vi "LoadCellDAQ.vi"(8 "error in (no error)":errorcluster, 9 "Message Notifiers":T1, 10 "UI Queue":refnum<queue>, 11 "Logging Queue":refnum<queue>) -> (0 "error out":errorcluster)   [LabVIEW 2018]
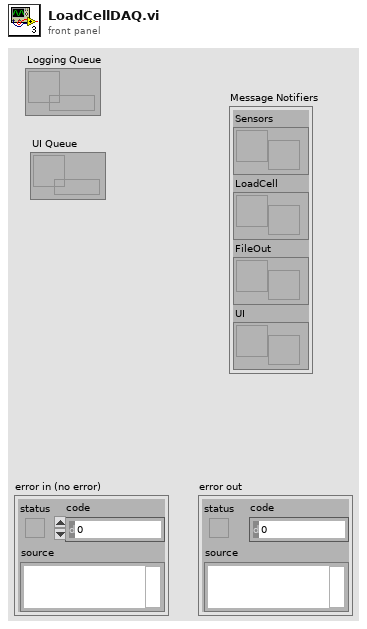
[diagram p1: front panel]
types:
  T1 = cluster{"Sensors":refnum<notifier>, "LoadCell":refnum<notifier>, "FileOut":refnum<notifier>, "UI":refnum<notifier>}
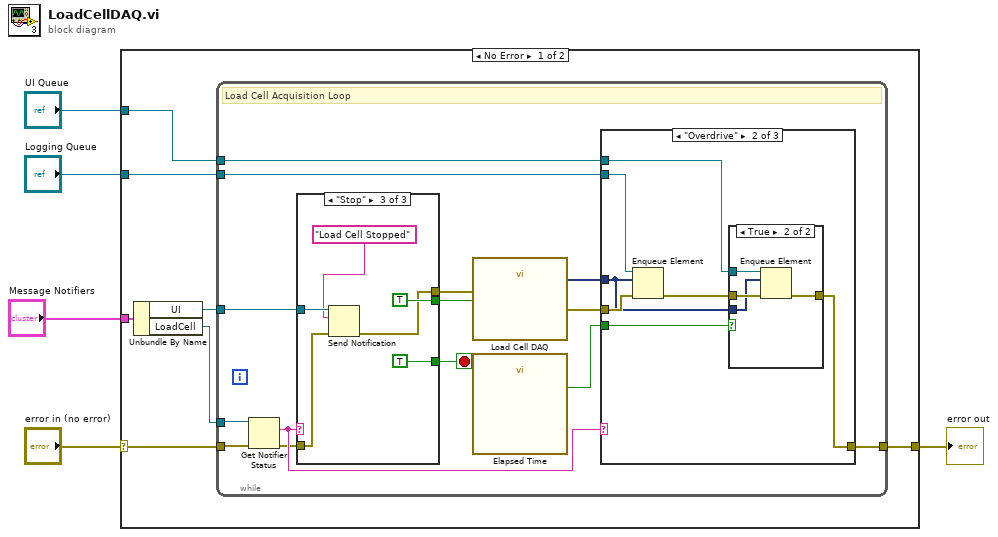
[diagram p0: block diagram]
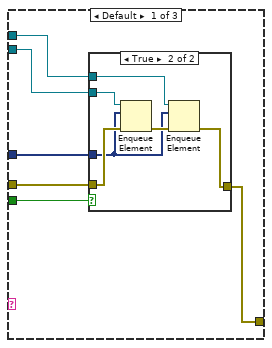
[diagram p2: hidden frame]
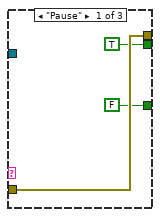
[diagram p6: hidden frame]
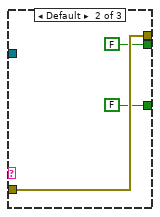
[diagram p7: hidden frame]
diagram:
  n1 = case shown="No Error" "error in (no error)" {
    selector: "error in (no error)" -> [w10 w65]
    tunnel: "Message Notifiers" -> [w12 _]
    tunnel: [w6 w65] -> w4
    tunnel: "Logging Queue" -> [w8 _]
    tunnel: "UI Queue" -> [w7 _]
    frame No Error {
      n2 = Unbundle By Name(w12) -> ("UI"=w11:refnum<notifier>, "LoadCell"=w9:refnum<notifier>)
      n3 = while {
        tunnel: w11 -> [w23]
        tunnel: w10 -> [w13]
        tunnel: w9 -> [w14]
        tunnel: w8 -> [w19]
        tunnel: w7 -> [w18]
        tunnel: [w21] -> w6
        stop <- w24 stop-if-true
        # "Load Cell Acquisition Loop"
        n4 = Get Notifier Status(notifier=w14, error in (no error)=w13) -> (current notification=w16:string, error out=w15:errorcluster)  [unwired: 3 out]
        n5 = case shown="\"Stop\"" w16 {
          tunnel: [TRUE FALSE TRUE] -> w26
          tunnel: [w55 w58 w60] -> w25
          tunnel: w15 -> [w55 w58 w61]
          tunnel: [FALSE FALSE TRUE] -> w24
          tunnel: w23 -> [_ _ w62]
          frame "Pause" {
          }
          frame Default {
          }
          frame "Stop" {
            n6 = Send Notification(notification="Load Cell Stopped", notifier=w62, error in (no error)=w61) -> (error out=w60:errorcluster)  [unwired: 1 out]
          }
        }
        n7 = call "Load Cell DAQ"("error in"=w25, "stop (F)"=w26) -> ("data"=w22:dynamicdata, "error out"=w20:errorcluster)  [unwired: 14 in, 2 out]
        n8 = call "Elapsed Time"() -> ("Time has Elapsed"=w17:bool)  [unwired: 12 in, 7 out]
        n9 = case shown="\"Overdrive\"" w16 {
          tunnel: w22 -> [w31 w41 _]
          tunnel: [w32 w42 w52] -> w21
          tunnel: w20 -> [w30 w46 w52]
          tunnel: w19 -> [w29 w45 _]
          tunnel: w18 -> [w28 w44 _]
          tunnel: w17 -> [w27 w40 _]
          frame Default {
            n10 = case shown="True" w27 {
              tunnel: w28 -> [_ w39]
              tunnel: w30 -> [w33 w36]
              tunnel: [w33 w38] -> w32
              tunnel: w31 -> [_ w34]
              tunnel: w29 -> [_ w35]
              frame False {
              }
              frame True {
                n11 = Enqueue Element(queue=w35, element=w34, error in (no error)=w36) -> (error out=w37:errorcluster)  [unwired: 1 in, 2 out]
                n12 = Enqueue Element(queue=w39, element=w34, error in (no error)=w37) -> (error out=w38:errorcluster)  [unwired: 1 in, 2 out]
              }
            }
          }
          frame "Overdrive" {
            n13 = Enqueue Element(queue=w45, element=w41, error in (no error)=w46) -> (error out=w43:errorcluster)  [unwired: 1 in, 2 out]
            n14 = case shown="True" w40 {
              tunnel: w44 -> [_ w51]
              tunnel: w43 -> [w47 w50]
              tunnel: [w47 w49] -> w42
              tunnel: w41 -> [_ w48]
              frame False {
              }
              frame True {
                n15 = Enqueue Element(queue=w51, element=w48, error in (no error)=w50) -> (error out=w49:errorcluster)  [unwired: 1 in, 2 out]
              }
            }
          }
          frame "Pause", "Stop" {
          }
        }
      }
    }
    frame Error {
    }
  }
  "error out" <- w4
